vi "apostrophe sanitizer.vi"(8 "error in (no error)":errorcluster, 9 "result from db":string, 11 "imput to db":string) -> (0 "error out":errorcluster, 1 "fixed result from db":string, 3 "fixed imput to db":string)   [LabVIEW 2012]
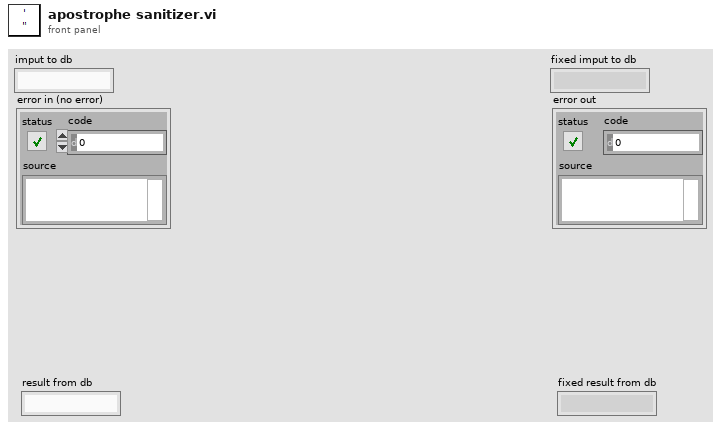
[diagram p1: front panel]
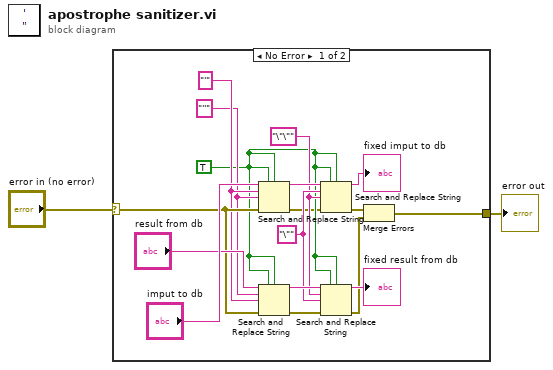
[diagram p0: block diagram]
diagram:
  n1 = case shown="No Error" "error in (no error)" {
    selector: "error in (no error)" -> [w17 w20]
    tunnel: [w16 w20] -> w1
    frame No Error {
      w6 = "\"\"" ("replace string (\"\")")
      w7 = "\"" ("search string")
      w14 = "''" ("replace string (\"\")")
      w15 = "'" ("search string")
      w5 = TRUE ("replace all? (F)")
      n2 = Search and Replace String(replace all?=w5, case sensitive?=w5, input string="imput to db", search string=w15, replace string=w14, error in=w17) -> (result string=w13:string, error out=w4:errorcluster)  [unwired: 2 in, 2 out]
      n3 = Search and Replace String(replace all?=w5, case sensitive?=w5, input string="result from db", search string=w14, replace string=w15, error in=w17) -> (result string=w11:string, error out=w9:errorcluster)  [unwired: 2 in, 2 out]
      n4 = Search and Replace String(replace all?=w5, case sensitive?=w5, input string=w13, search string=w7, replace string=w6, error in=w4) -> (result string=→"fixed imput to db":string, error out=w3:errorcluster)  [unwired: 2 in, 2 out]
      n5 = Search and Replace String(replace all?=w5, case sensitive?=w5, input string=w11, search string=w6, replace string=w7, error in=w9) -> (result string=→"fixed result from db":string, error out=w8:errorcluster)  [unwired: 2 in, 2 out]
      n6 = Merge Errors(w3, w8) -> (w16:errorcluster)
    }
    frame Error {
    }
  }
  "error out" <- w1
